vi "Copy file to network and group server.vi"(11 "File path in":path) -> ()   [LabVIEW 2013]
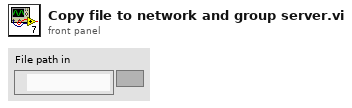
[diagram p1: front panel]
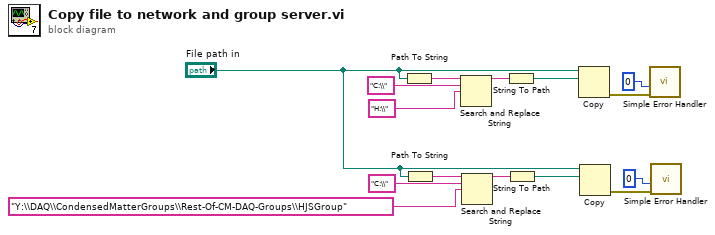
[diagram p0: block diagram]
diagram:
  n1 = Path To String(path="File path in") -> (string=w13:string)
  n2 = Path To String(path="File path in") -> (string=w8:string)
  n3 = Search and Replace String(input string=w13, search string="C:\\", replace string="H:\\") -> (result string=w15:string)  [unwired: 5 in, 3 out]
  n4 = Search and Replace String(input string=w8, search string="C:\\", replace string="Y:\\DAQ\\CondensedMatterGroups\\Rest-Of-CM-DAQ-Groups\\HJSGroup") -> (result string=w10:string)  [unwired: 5 in, 3 out]
  n5 = String To Path(string=w15) -> (path=w14:path)
  n6 = String To Path(string=w10) -> (path=w9:path)
  n7 = Copy(10:w14, 11:"File path in") -> (0:w4:errorcluster)  [unwired: 3 in, 2 out]
  n8 = Copy(10:w9, 11:"File path in") -> (0:w2:errorcluster)  [unwired: 3 in, 2 out]
  n9 = call <vilib>:"Simple Error Handler.vi"("type of dialog (OK msg:1)"=0, "error in (no error)"=w4) -> ()  [unwired: 3 in, 5 out]
  n10 = call <vilib>:"Simple Error Handler.vi"("type of dialog (OK msg:1)"=0, "error in (no error)"=w2) -> ()  [unwired: 3 in, 5 out]
